vi "Output_Curve.vi"(0 "File Path":path, 1 "V_DS Start":dbl=-0.7 format="%#.3g", 2 "V_DS Finish":dbl=3.0 format="%#.3g", 3 "V_DS Step Size":dbl=0.1 format="%#.3g", 4 "Preread delay (ms)":dbl=5000.0 format="%.2f", 5 "Delay between \naverages (ms)":dbl=200.0 format="%#.3f", 6 "Keithley 237 GPIB address":string="17", 7 "Software Averages":i16=5, 8 "VISA resource name":refnum<visa-resource-name>="GPIB0::24::INSTR", 9 "First bias settle (ms)":dbl=2000.0 format="%#.2f", 10 "V_G":dbl=0.1 format="%#_13g", 11 "Current Compliance\nLimit (A) Ke2400":dbl=1.0 format="%#.3e", 12 "Dimensions":T1(ring), 17 "Voltage Compliance Limit 237 (V)":dbl=10.0 format="%#.3f", 18 "Current Compliance\nLimit 237 (A)":dbl=0.1 format="%#.3f") -> ()   [LabVIEW 2018]
uses:
  <vilib>/Utility/file.llb/Write Delimited Spreadsheet (string).vi
  Instance           1 16Saved   JV curve .vi
  <userlib>/KE237.LLB/Keith 237 Operate/Standby.vi
  <instrlib>/Keithley 24XX/Public/Data/Read (Single Point).vi
  <vilib>/Analysis/NI_AALBase.lvlib
  <instrlib>/Keithley 24XX/Keithley 24XX.lvlib
panel:
  out "Keithley 2400":cluster{dbl[], dbl[]}(graph)={[-2.0, -1.9, -1.8, -1.7, -1.6, -1.5], [-6.6965744e-11, -6.7804984e-11, -6.685451799999999e-11, -6.6450076e-11, -6.5125542e-11, -6.7339852e-11]}
  out "I_G":dbl=-6.642986e-11 format="%.2e"
  in  "Autozero?":u16(ring) items=["On", "Off", "Once"]
  in  "Measurement Speed (1 PLC)":dbl=1.0 format="%.2g"
  in  "Manual Range (Max I)":dbl=1.0
  in  "Enable Meas Auto Range":bool=TRUE
  in  "Source Mode":u16(ring) items=["Voltage", "Current"]
  in  "Return Sweep?":bool
  out "I_DS":dbl=-1.38e-12 format="%.2e"
  out "Outputfile":path=path "C:/DATA/Mark Ziffer/test10"
  in  "Abort Scan":bool=TRUE
  out "V_DS":dbl=-1.5 format="%#.2f"
  out "Keithley 237":cluster{dbl[], dbl[]}(graph)={[-2.0, -1.9, -1.8, -1.7, -1.6, -1.5], [-6.720000000000001e-13, -2.18e-13, -2.7599999999999993e-13, -8.999999999999998e-14, -1.3999999999999998e-13, -1.3800000000000002e-13]}
  # "Output Curve\nbased on  EL_photocurrent_JV.vi for controlling 2 Ketthleys\n\n9/2017 MZ"
  # "Software Settings"
  # "Ke237 Settings"
  # "Ke2400 Settings"
  # "Notes for IV Scan\n\n2010.07.06 - add absolute value plotter to look at log-scale current\n2010.01.07 - Modified file headers for distinguihing when imported to Igor Pro - the prefix of each header will be the file name.\n2009.01.15 - I updated the code to run on the VISA driver convention. I also modified the file saving and the option to set the\n                      graph display.\n2008.12.01 - I fixed an issue with calculations of J. It was mis-wired to divide current by wavelength, rather than active area.  BM\n\n=========================\nI added the functionality to calculate the fill factor, rectification ratio, short circuit current density, and open circuit voltage. \nAdditionally, current density (mA/cm^2) is reported in the plot window and column B of the data file, and the current (A) has been \nmoved to column C. Open circuit voltage is linearly interpolated. The max power point (mpp) for calculating fill factor is taken as \nthe data point with the highest I-V product, so this makes it only as accurate as your voltage step size, but should be fine for a decent \ndevice on the 50 mV default step size.\n\nIf you know how to use the previous versions of IV scan, \nmake sure you set these parameters before you scan:\n1) Recftification Ratio Bias - this is the +/- bias value you wish to record a rectification ratio at.\n2) Effective Area - this is the area in cm^2 of the diode mask (photoactive area) when measuring under illumination or the measured \n     area of the electrode overlap when measured in dark (regular active area).\n3) Do you want to record a separate data file for the calculated characteristics? If so, make sure the switch is on.\n\nAs of today, I couldn't figure out how to append the computed characteristics to the I-V file without experiencing formating issues, so\nI opted to just create a separate file if you want to save that info. Feel free to fix this if you know how. Check tab 3 > tab 2 > tab 9 in the\nblock diagram.\n\n2008-04-15\nB MacLeod"
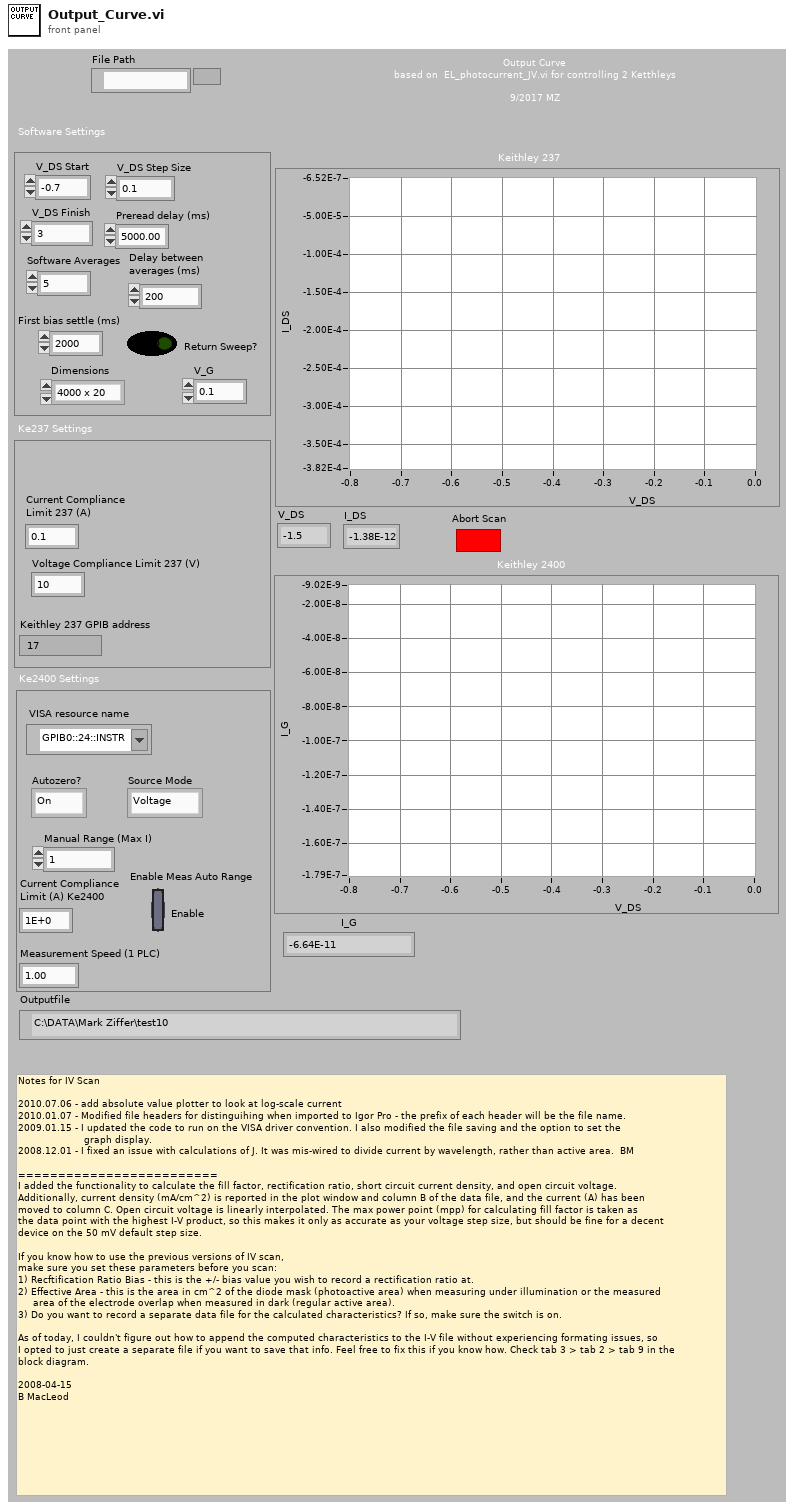
[diagram p1: front panel]
types:
  T1 = enum16{"4000 x 20", "2000 x 20", "1000 x 20", "800 x 20", "400 x 20", "200 x 20", "100 x 20"}
  T2 = cluster{"error":bool, "code":i32, "source":string}
  T3 = cluster{"source value":string, "measure value":string, "delay value (sec)":string, "time value (sec)":string}[]
  T4 = cluster{"source value":dbl, "measure value":dbl, "delay value (sec)":dbl, "time value (sec)":dbl}[]
  T5 = cluster{"[0]":cluster{"source value":dbl, "measure value":dbl, "delay value (sec)":dbl, "time value (sec)":dbl}, "[1]":cluster{"source value":dbl, "measure value":dbl, "delay value (sec)":dbl, "time value (sec)":dbl}, "[2]":cluster{"source value":dbl, "measure value":dbl, "delay value (sec)":dbl, "time value (sec)":dbl}, "[3]":cluster{"source value":dbl, "measure value":dbl, "delay value (sec)":dbl, "time value (sec)":dbl}, "[4]":cluster{"source value":dbl, "measure value":dbl, "delay value (sec)":dbl, "time value (sec)":dbl}, "[5]":cluster{"source value":dbl, "measure value":dbl, "delay value (sec)":dbl, "time value (sec)":dbl}, "[6]":cluster{"source value":dbl, "measure value":dbl, "delay value (sec)":dbl, "time value (sec)":dbl}, "[7]":cluster{"source value":dbl, "measure value":dbl, "delay value (sec)":dbl, "time value (sec)":dbl}, "[8]":cluster{"source value":dbl, "measure value":dbl, "delay value (sec)":dbl, "time value (sec)":dbl}}
  T6 = cluster{"source value":dbl, "measure value":dbl, "delay value (sec)":dbl, "time value (sec)":dbl}
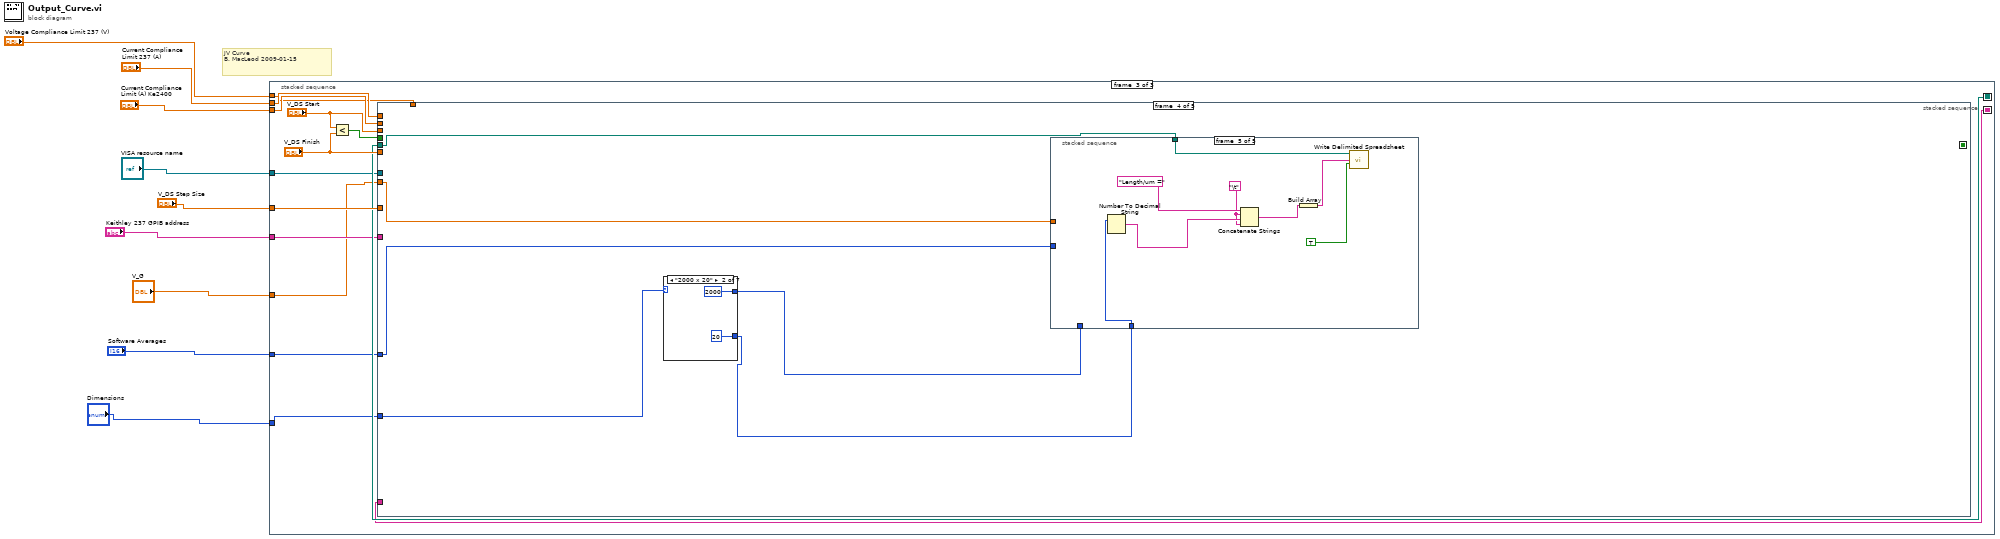
[diagram p0: block diagram]
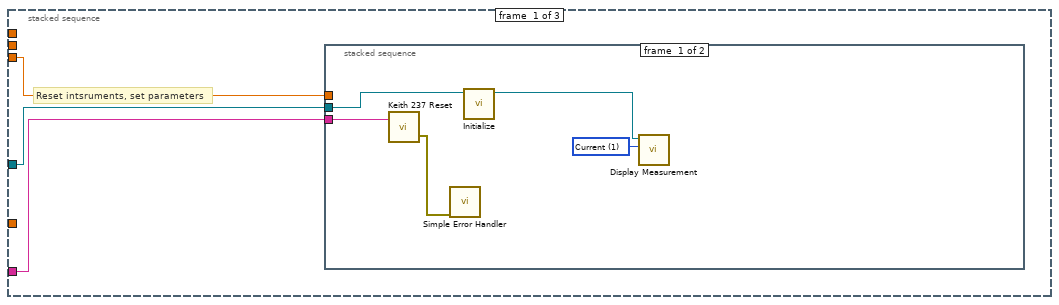
[diagram p2: hidden frame]
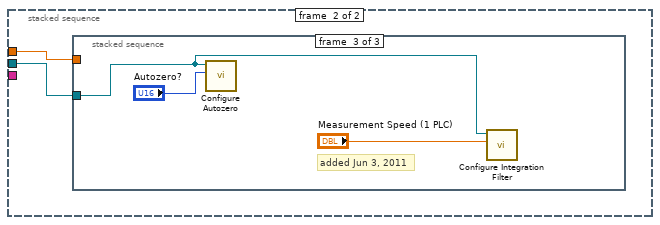
[diagram p3: hidden frame]
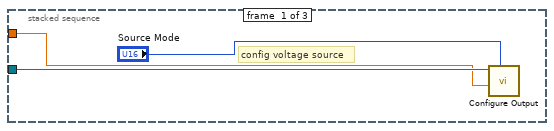
[diagram p4: hidden frame]
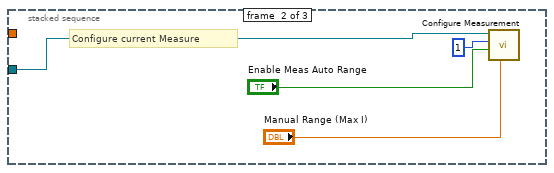
[diagram p5: hidden frame]
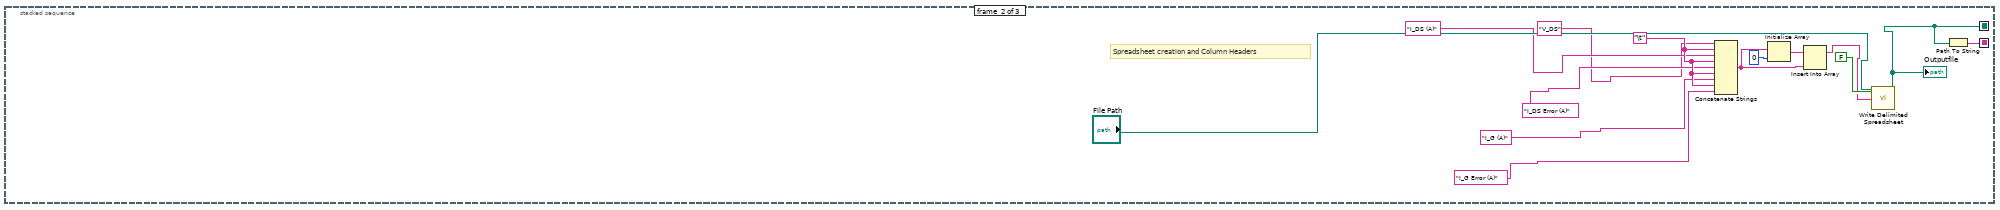
[diagram p6: hidden frame]
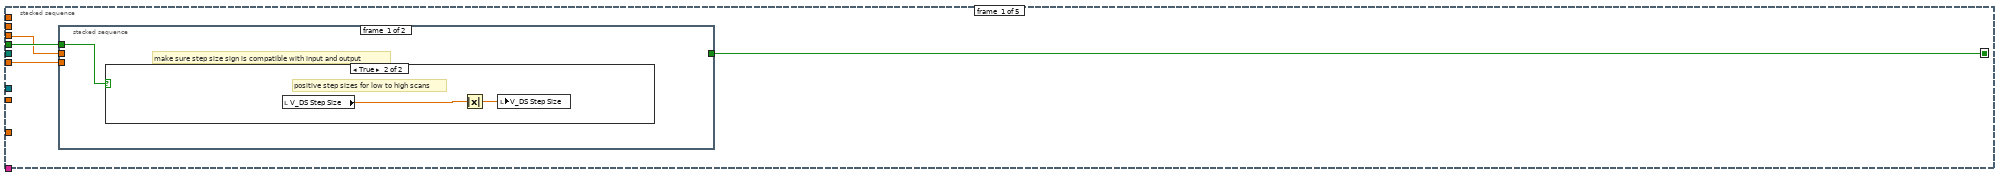
[diagram p7: hidden frame]
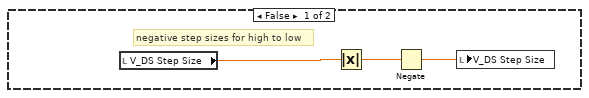
[diagram p8: hidden frame]
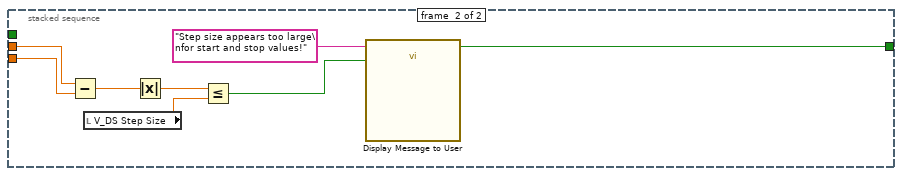
[diagram p9: hidden frame]
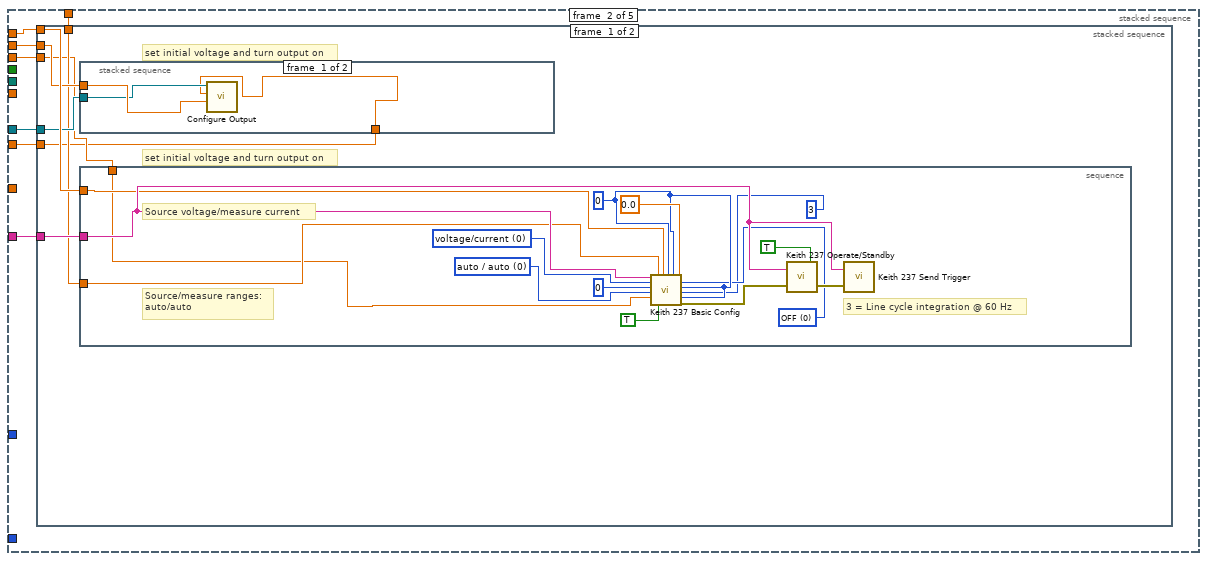
[diagram p10: hidden frame]
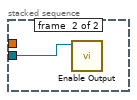
[diagram p11: hidden frame]
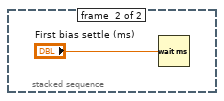
[diagram p12: hidden frame]
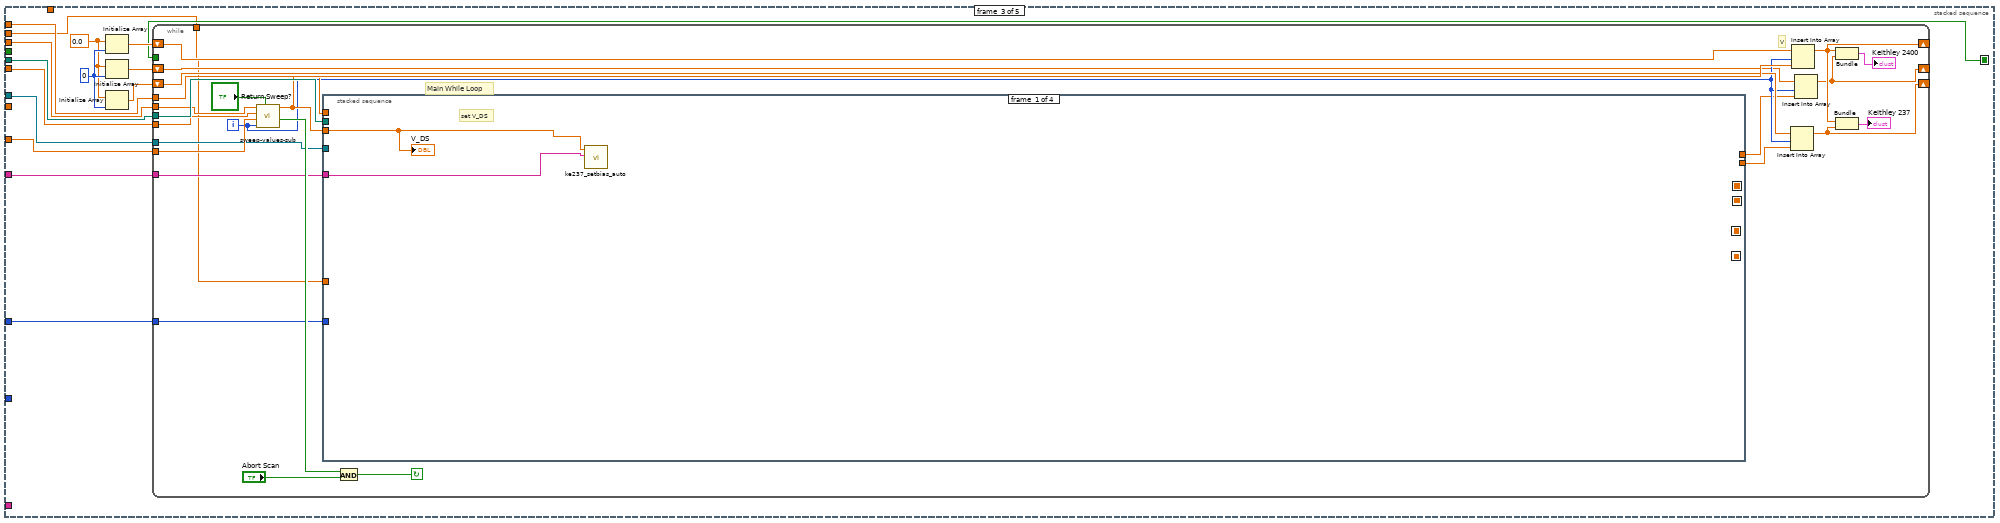
[diagram p13: hidden frame]
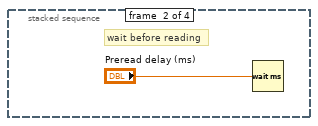
[diagram p14: hidden frame]
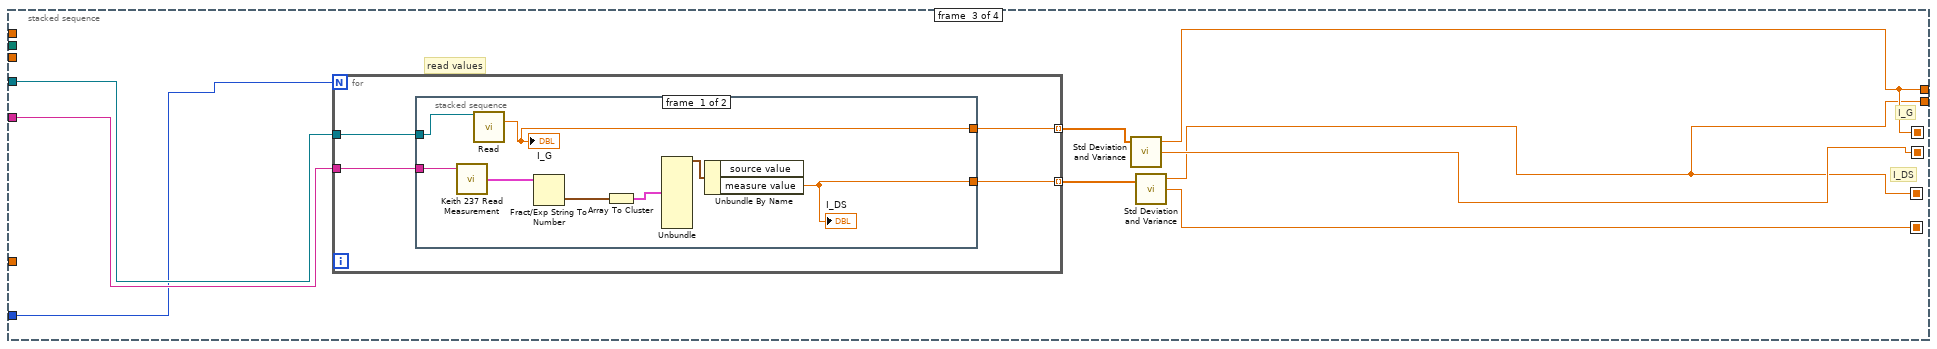
[diagram p15: hidden frame]
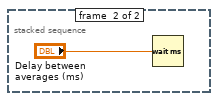
[diagram p16: hidden frame]
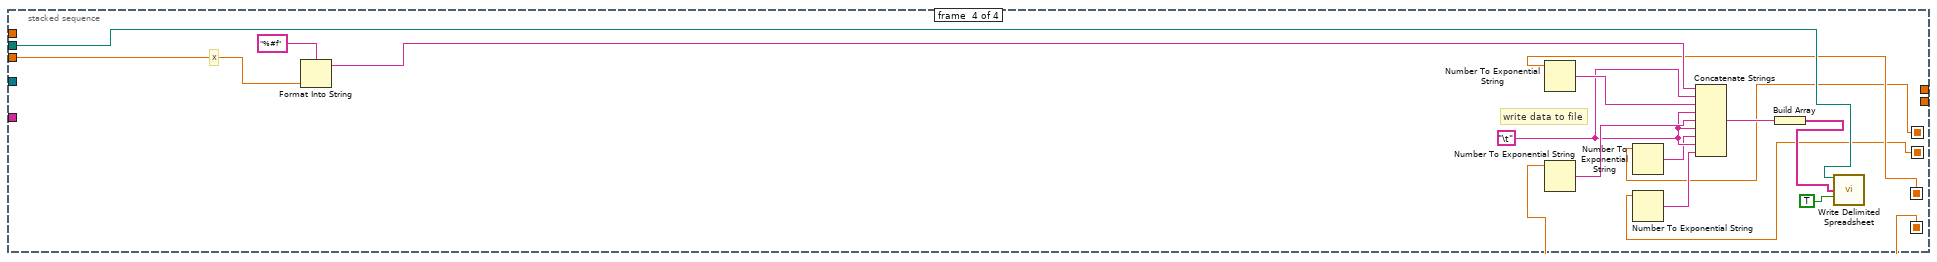
[diagram p17: hidden frame]
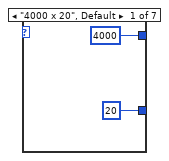
[diagram p18: hidden frame]
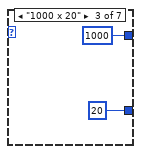
[diagram p19: hidden frame]
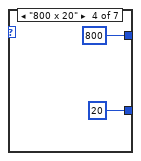
[diagram p20: hidden frame]
diagram:
  # "JV Curve\nB. MacLeod 2009-01-15"
  n1 = stacked-sequence {
    seq-local: [_ w36 _] -> [_ _ w53]
    seq-local: [_ w43 _] -> [_ _ w52]
    tunnel: "V_DS Step Size" -> [_ _ w54]
    tunnel: "Current Compliance\nLimit 237 (A)" -> [_ _ w51]
    tunnel: "Voltage Compliance Limit 237 (V)" -> [_ _ w47]
    tunnel: "Keithley 237 GPIB address" -> [w12 _ w50]
    tunnel: "VISA resource name" -> [w11 _ w49]
    tunnel: "Current Compliance\nLimit (A) Ke2400" -> [w10 _ w48]
    tunnel: "V_G" -> [_ _ w46]
    tunnel: "Software Averages" -> [_ _ w45]
    tunnel: "Dimensions" -> [_ _ w44]
    frame #0 {
      # "Reset intsruments, set parameters"
      n2 = stacked-sequence {
        tunnel: w12 -> [w16 _]
        tunnel: w11 -> [w15 w19]
        tunnel: w10 -> [_ w18]
        frame #0 {
          w14 = u16 1 items=["Voltage", "Current", "Resistance"] ("Displayed Measurement (0: Voltage)")
          n3 = call <userlib>:"Keith 237 Reset.vi"("GPIB address"=w16) -> ("error out"=w17:T2)  [unwired: 1 in]
          n4 = call <vilib>:"Simple Error Handler.vi"("error in (no error)"=w17) -> ()  [unwired: 1 in, 8 out]
          n5 = call <instrlib>:"Initialize.vi"("VISA resource name"=w15) -> ("VISA resource name out"=w13:refnum<visa-resource-name>)  [unwired: 9 in, 1 out]
          n6 = call <instrlib>:"Display Measurement.vi"("Displayed Measurement (0: Voltage)"=w14, "VISA resource name"=w13) -> ()  [unwired: 8 in, 2 out]
        }
        frame #1 {
          n7 = stacked-sequence {
            tunnel: w19 -> [w21 w23 w27]
            tunnel: w18 -> [w20 _ _]
            frame #0 {
              # "config voltage source"
              n8 = call <instrlib>:"Configure Output.vi"("Source Mode  (0: Voltage)"="Source Mode", "Compliance  Level (0.1)"=w20, "VISA resource name"=w21) -> ()  [unwired: 3 in, 6 out]
            }
            frame #1 {
              # "Configure current Measure"
              n9 = call <instrlib>:"Configure Measurement.vi"("Manual Range (1.0)"="Manual Range (Max I)", "Enable Auto Range (T:Enable)"="Enable Meas Auto Range", "Function (0: Volts)"=1, "VISA resource name"=w23) -> ()  [unwired: 1 in, 7 out]
            }
            frame #2 {
              # "added Jun 3, 2011"
              n10 = call <instrlib>:"Configure Autozero.vi"("Autozero  (0: On)"="Autozero?", "VISA resource name"=w27) -> ()  [unwired: 1 in, 9 out]
              n11 = call <instrlib>:"Configure Integration Filter.vi"("Measurement Speed (1 PLC)"="Measurement Speed (1 PLC)", "VISA resource name"=w27) -> ()  [unwired: 8 in, 2 out]
            }
          }
        }
      }
    }
    frame #1 {
      w39 = "\t"
      # "Spreadsheet creation and Column Headers"
      n12 = Concatenate Strings("V_DS", w39, "I_DS (A)", w39, "I_DS Error (A)", w39, "I_G (A)", w39, "I_G Error (A)" ("string")) -> (w41:string)
      n13 = Initialize Array(w41, 0 ("dimension size")) -> (w40:string[])
      n14 = Insert Into Array(array=w40, new element=w41) -> (w37:string[])  [unwired: 1 in]
      n15 = call-poly <vilib>:"Write Delimited Spreadsheet.vi"("file path (dialog if empty)"="File Path", "1D data"=w37, "transpose? (no:F)"=FALSE ("append to file? (new file:F)")) -> ("new file path (Not A Path if cancelled)"=w36:path)  [unwired: 11 in, 1 out]
      "Outputfile" <- w36
      n16 = Path To String(path=w36) -> (string=w43:string)
    }
    frame #2 {
      n17 = Less?(x="V_DS Start", y="V_DS Finish") -> (x < y?=w55:bool)
      n18 = stacked-sequence {
        seq-local: [w58 _ _ _ _] -> [_ _ w117 _ _]
        tunnel: w55 -> [w61 _ _ _ _]
        tunnel: "V_DS Start" -> [w60 w77 w123 _ _]
        tunnel: "V_DS Finish" -> [w59 _ w124 _ _]
        tunnel: w54 -> [_ _ w122 _ _]
        tunnel: w53 -> [_ _ w121 w194 _]
        tunnel: w52 -> [_ _ _ _ _]
        tunnel: w51 -> [_ w82 w118 _ _]
        tunnel: w50 -> [_ w81 w116 _ w251]
        tunnel: w49 -> [_ w79 w115 _ w250]
        tunnel: w48 -> [_ w80 w111 _ _]
        tunnel: w47 -> [_ w78 _ _ _]
        tunnel: w46 -> [_ w76 _ w196 _]
        tunnel: w45 -> [_ _ w110 w195 _]
        tunnel: w44 -> [_ _ _ w193 _]
        frame #0 {
          n19 = stacked-sequence {
            tunnel: w61 -> [w62 _]
            tunnel: w60 -> [_ w75]
            tunnel: w59 -> [_ w74]
            tunnel: [_ w68] -> w58
            frame #0 {
              # "make sure step size sign is compatible with input and output"
              n20 = case shown="True" w62 {
                frame False {
                  # "negative step sizes for high to low"
                  n21 = local read "V_DS Step Size"() -> (w65:dbl)
                  n22 = Absolute Value(x=w65) -> (abs(x)=w64:dbl)
                  n23 = Negate(x=w64) -> (-x=w63:dbl)
                  n24 = local write "V_DS Step Size"(w63) -> ()
                }
                frame True {
                  # "positive step sizes for low to high scans"
                  n25 = local read "V_DS Step Size"() -> (w67:dbl)
                  n26 = Absolute Value(x=w67) -> (abs(x)=w66:dbl)
                  n27 = local write "V_DS Step Size"(w66) -> ()
                }
              }
            }
            frame #1 {
              n28 = Subtract(x=w75, y=w74) -> (x-y=w73:dbl)
              n29 = local read "V_DS Step Size"() -> (w71:dbl)
              n30 = Absolute Value(x=w73) -> (abs(x)=w72:dbl)
              n31 = Less Or Equal?(x=w72, y=w71) -> (x <= y?=w69:bool)
              n32 = call "Display Message to User"("Enable"=w69, "Message"="Step size appears too large\nfor start and stop values!") -> ("OK"=w68:bool)  [unwired: 1 in, 8 out]
            }
          }
        }
        frame #1 {
          n33 = stacked-sequence {
            tunnel: w82 -> [w89 _]
            tunnel: w81 -> [w88 _]
            tunnel: w80 -> [w87 _]
            tunnel: w79 -> [w86 _]
            tunnel: w78 -> [w85 _]
            tunnel: w77 -> [w84 _]
            tunnel: w76 -> [w83 _]
            frame #0 {
              # "set initial voltage and turn output on"
              # "set initial voltage and turn output on"
              n34 = stacked-sequence {
                tunnel: w87 -> [w92 _]
                tunnel: w86 -> [w91 w93]
                tunnel: w83 -> [w90 _]
                frame #0 {
                  n35 = call <instrlib>:"Configure Output.vi"("Compliance  Level (0.1)"=w92, "Output Level (0)"=w90, "VISA resource name"=w91) -> ()  [unwired: 3 in, 6 out]
                }
                frame #1 {
                  n36 = call <instrlib>:"Enable Output.vi"("VISA resource name"=w93) -> ()  [unwired: 2 in, 9 out]
                }
              }
              n37 = stacked-sequence {
                tunnel: w89 -> [w97]
                tunnel: w88 -> [w99]
                tunnel: w85 -> [w96]
                tunnel: w84 -> [w94]
                frame #0 {
                  w98 = u16 0 items=["OFF", "ON"] ("default delay (on:1)")
                  w100 = u16 0 items=["auto / auto", "1 nA / 1.1 V", "10 nA / 11 V", "100 nA / 110 V", "0.001 mA / 1100 V", "0.01 mA / 1100 V", "0.1 mA / 1100 V", "1 mA / 1100 V", "10 mA / 1100 V", "100 mA / 1100 V"] ("source range\nI source / V source (auto:0)")
                  w101 = u16 0 items=["voltage/current", "current/voltage"] ("source/measure (V/I:0)")
                  w103 = u16 0
                  # "3 = Line cycle integration @ 60 Hz"
                  # "Source/measure ranges:\nauto/auto"
                  # "Source voltage/measure current"
                  n38 = call <userlib>:"Keith 237 Basic Config.vi"("GPIB address"=w99, "source/measure (V/I:0)"=w101, "function (DC:0)"=u16 0, "source range\nI source / V source (auto:0)"=w100, "source level"=w94, "voltage \ncompliance level"=w96, "1100 V range (disabled:F)"=TRUE, "current \ncompliance level"=w97, "compliance/\nmeasurement range (auto:0)"=w103, "suppression (off:0)"=w103, "DC delay (sec)"=0.0, "default delay (on:1)"=w98, "filter (disabled:0)"=w103, "integration time (medium:1)"=u16 3, "sense (local:0)"=w103) -> ("error out"=w108:T2)  [unwired: 4 in]
                  n39 = call "Keith 237 Operate/Standby.vi"("source"=TRUE, "error in"=w108, "GPIB address"=w99) -> ("error out"=w106:T2)
                  n40 = call <userlib>:"Keith 237 Send Trigger.vi"("GPIB address"=w99, "error in"=w106) -> ()  [unwired: 1 out]
                }
              }
            }
            frame #1 {
              n41 = Wait (ms)(milliseconds to wait="First bias settle (ms)") -> ()  [unwired: 1 out]
            }
          }
        }
        frame #2 {
          w114 = 0
          w113 = 0.0
          n42 = Initialize Array(w113, w114) -> (w120:dbl[])
          n43 = Initialize Array(w113, w114) -> (w112:dbl[])
          n44 = Initialize Array(w113, w114) -> (w119:dbl[])
          n45 = while {
            shift-left: w119 -> [w145]
            shift-right: [w133] -> _
            shift-left: w120 -> [w146]
            shift-right: [w136] -> _
            tunnel: w121 -> [w148]
            tunnel: w122 -> [w144]
            tunnel: w123 -> [w143]
            tunnel: w124 -> [w142]
            tunnel: w118 -> [w140]
            tunnel: w117 -> [_]
            shift-right: [w132] -> _
            shift-left: w112 -> [w128]
            tunnel: w116 -> [w131]
            tunnel: w115 -> [w130]
            tunnel: w111 -> [w126]
            tunnel: w110 -> [w125]
            i -> [w134]
            stop <- w138 continue-if-true
            # "Main While Loop"
            # "V"
            n46 = call "sweep-values-sub.vi"("Forward/Reverse"="Return Sweep?", "Point Number"=w134, "Step Size"=w144, "Sweep Stop"=w142, "Sweep Start"=w143) -> ("Active"=w139:bool, "Output"=w147:dbl)  [unwired: 2 out]
            n47 = stacked-sequence {
              seq-local: [_ _ w161 _] -> [_ _ _ w177]
              seq-local: [_ _ w155 _] -> [_ _ _ w178]
              seq-local: [_ _ w157 _] -> [_ _ _ w176]
              seq-local: [_ _ w156 _] -> [_ _ _ w175]
              tunnel: [_ _ w155 _] -> w135
              tunnel: w147 -> [w150 _ _ w189]
              tunnel: w148 -> [_ _ _ w180]
              tunnel: w140 -> [_ _ _ _]
              tunnel: w131 -> [w151 _ w159 _]
              tunnel: w130 -> [_ _ w158 _]
              tunnel: [_ _ w157 _] -> w129
              tunnel: w126 -> [_ _ _ _]
              tunnel: w125 -> [_ _ w154 _]
              frame #0 {
                # "set V_DS"
                n48 = call "ke237_setbias_auto.vi"("GPIB address"=w151, "source level"=w150) -> ()  [unwired: 10 in]
                "V_DS" <- w150
              }
              frame #1 {
                # "wait before reading"
                n49 = Wait (ms)(milliseconds to wait="Preread delay (ms)") -> ()  [unwired: 1 out]
              }
              frame #2 {
                # "I_DS"
                # "I_G"
                # "read values"
                n50 = for {
                  N: w154 -> [_]
                  tunnel: [w165] -> w160 mode=indexing
                  tunnel: w159 -> [w164]
                  tunnel: w158 -> [w163]
                  tunnel: [w162] -> w153 mode=indexing
                  n51 = stacked-sequence {
                    tunnel: [w170 _] -> w165
                    tunnel: w164 -> [w168 _]
                    tunnel: w163 -> [w167 _]
                    tunnel: [w166 _] -> w162
                    frame #0 {
                      n52 = call <userlib>:"Keith 237 Read Measurement.vi"("GPIB address"=w168) -> ("display"=w173:T3)  [unwired: 1 in, 3 out]
                      n53 = call-poly <instrlib>:"Read.vi"("VISA resource name"=w167) -> ("Current"=w166:sgl)  [unwired: 8 in, 6 out]
                      "I_G" <- w166
                      n54 = Fract/Exp String To Number(string=w173) -> (number=w169:T4)  [unwired: 3 in, 1 out]
                      n55 = Array To Cluster(array=w169) -> (cluster=w172:T5)
                      n56 = Unbundle(w172) -> ("[0]"=w171:T6)  [unwired: 8 out]
                      n57 = Unbundle By Name(w171) -> ("measure value"=w170:dbl)  [unwired: 1 out]
                      "I_DS" <- w170
                    }
                    frame #1 {
                      n58 = Wait (ms)(milliseconds to wait="Delay between \naverages (ms)") -> ()  [unwired: 1 out]
                    }
                  }
                }
                n59 = call <vilib>:"Std Deviation and Variance.vi"("X"=w153) -> ("mean"=w157:dbl, "standard deviation"=w156:dbl)  [unwired: 1 in, 1 out]
                n60 = call <vilib>:"Std Deviation and Variance.vi"("X"=w160) -> ("mean"=w155:dbl, "standard deviation"=w161:dbl)  [unwired: 1 in, 1 out]
              }
              frame #3 {
                w184 = "\t"
                # "write data to file"
                # "X"
                n61 = Format Into String(format string="%#f", w189) -> (resulting string=w187:string)  [unwired: 2 in, 1 out]
                n62 = Number To Exponential String(number=w178) -> (E-format string=w190:string)  [unwired: 3 out]
                n63 = Number To Exponential String(number=w177) -> (E-format string=w186:string)  [unwired: 3 out]
                n64 = Number To Exponential String(number=w176) -> (E-format string=w183:string)  [unwired: 3 out]
                n65 = Number To Exponential String(number=w175) -> (E-format string=w182:string)  [unwired: 3 out]
                n66 = Concatenate Strings(w187, w184, w190, w184, w186, w184, w183, w184, w182) -> (w185:string)
                n67 = Build Array(w185) -> (w181:string[])
                n68 = call-poly <vilib>:"Write Delimited Spreadsheet.vi"("file path (dialog if empty)"=w180, "1D data"=w181, "append to file? (new file:F)"=TRUE) -> ()  [unwired: 11 in, 2 out]
              }
            }
            n69 = Compound Arithmetic op=AND(w139, "Abort Scan") -> (w138:bool)
            n70 = Insert Into Array(array=w145, index=w134, new element=w135) -> (w133:dbl[])
            n71 = Insert Into Array(array=w146, index=w134, new element=w147) -> (w136:dbl[])
            n72 = Insert Into Array(array=w128, index=w134, new element=w129) -> (w132:dbl[])
            n73 = Bundle(w136, w132) -> (→"Keithley 2400":cluster{dbl[], dbl[]})  [unwired: 1 out]
            n74 = Bundle(w136, w133) -> (→"Keithley 237":cluster{dbl[], dbl[]})  [unwired: 1 out]
          }
        }
        frame #3 {
          n75 = case shown="\"2000 x 20\"" w193 {
            tunnel: [4000 2000 1000 800 400 200 100] -> w192
            tunnel: [20 20 20 20 20 20 20] -> w191
            frame "4000 x 20", Default {
            }
            frame "2000 x 20" {
            }
            frame "1000 x 20" {
            }
            frame "800 x 20" {
            }
            frame "400 x 20" {
            }
            frame "200 x 20" {
            }
            frame "100 x 20" {
            }
          }
          n76 = stacked-sequence {
            tunnel: w196 -> [_ w222 _ _ _]
            tunnel: w194 -> [w211 w220 w226 w234 w242]
            tunnel: w195 -> [_ _ w228 _ _]
            tunnel: w192 -> [_ _ _ w235 _]
            tunnel: w191 -> [_ _ _ _ w243]
            frame #0 {
              w216 = ""
              w215 = "\t"
              n77 = Concatenate Strings(w216, w215, w216, w215) -> (w212:string)
              n78 = Build Array(w212) -> (w214:string[])
              n79 = call-poly <vilib>:"Write Delimited Spreadsheet.vi"("file path (dialog if empty)"=w211, "1D data"=w214, "append to file? (new file:F)"=TRUE) -> ()  [unwired: 11 in, 2 out]
            }
            frame #1 {
              w223 = "\t"
              n80 = Number To Fractional String(number=w222, precision (6)=3) -> (F-format string=w221:string)  [unwired: 2 in]
              n81 = Concatenate Strings("V_G = ", w223, w221, w223) -> (w224:string)
              n82 = Build Array(w224) -> (w219:string[])
              n83 = call-poly <vilib>:"Write Delimited Spreadsheet.vi"("file path (dialog if empty)"=w220, "1D data"=w219, "append to file? (new file:F)"=TRUE) -> ()  [unwired: 11 in, 2 out]
            }
            frame #2 {
              w231 = "\t"
              n84 = Number To Decimal String(number=w228) -> (decimal integer string=w227:string)  [unwired: 1 in]
              n85 = Concatenate Strings("Number of Averages = ", w231, w227, w231) -> (w232:string)
              n86 = Build Array(w232) -> (w230:string[])
              n87 = call-poly <vilib>:"Write Delimited Spreadsheet.vi"("file path (dialog if empty)"=w226, "1D data"=w230, "append to file? (new file:F)"=TRUE) -> ()  [unwired: 11 in, 2 out]
            }
            frame #3 {
              w239 = "\t"
              n88 = Number To Decimal String(number=w235) -> (decimal integer string=w238:string)  [unwired: 1 in]
              n89 = Concatenate Strings("Width/um =", w239, w238, w239) -> (w237:string)
              n90 = Build Array(w237) -> (w236:string[])
              n91 = call-poly <vilib>:"Write Delimited Spreadsheet.vi"("file path (dialog if empty)"=w234, "1D data"=w236, "append to file? (new file:F)"=TRUE) -> ()  [unwired: 11 in, 2 out]
            }
            frame #4 {
              w244 = "\t"
              n92 = Number To Decimal String(number=w243) -> (decimal integer string=w247:string)  [unwired: 1 in]
              n93 = Concatenate Strings("Length/um =", w244, w247, w244) -> (w248:string)
              n94 = Build Array(w248) -> (w249:string[])
              n95 = call-poly <vilib>:"Write Delimited Spreadsheet.vi"("file path (dialog if empty)"=w242, "1D data"=w249, "append to file? (new file:F)"=TRUE) -> ()  [unwired: 11 in, 2 out]
            }
          }
        }
        frame #4 {
          # "reset instrument at end of sweep"
          n96 = call <instrlib>:"Reset.vi"("VISA resource name"=w250) -> ()  [unwired: 9 in, 2 out]
          n97 = call <userlib>:"Keith 237 Reset.vi"("GPIB address"=w251) -> ()  [unwired: 1 in, 1 out]
        }
      }
    }
  }
